vi "calculator.vi"() -> ()   [LabVIEW 2020]
panel:
  out "结果":string
  out "表达式":string
  in  "BACKPLACE":bool
  in  "C":bool
  in  "ln":bool
  in  "^":bool
  in  "tan":bool
  in  "cos":bool
  in  "sin":bool
  in  ")":bool
  in  "(":bool
  in  ".":bool
  in  "=":bool
  in  "0":bool
  in  "9":bool
  in  "8":bool
  in  "7":bool
  in  "6":bool
  in  "5":bool
  in  "4":bool
  in  "3":bool
  in  "2":bool
  in  "1":bool
  in  "÷":bool
  in  "×":bool
  in  "-":bool
  in  "+":bool
  # "科学计算器"
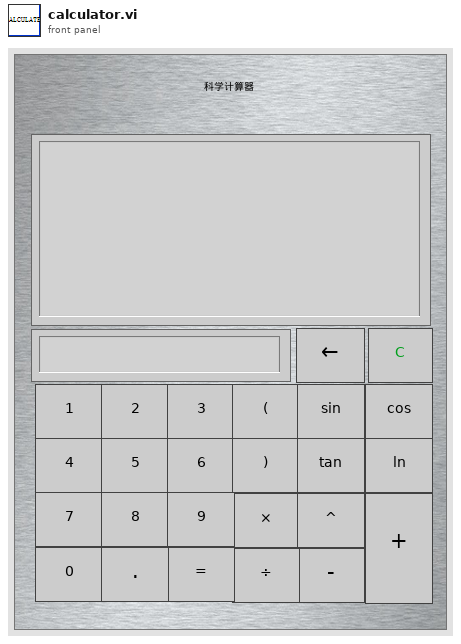
[diagram p1: front panel]
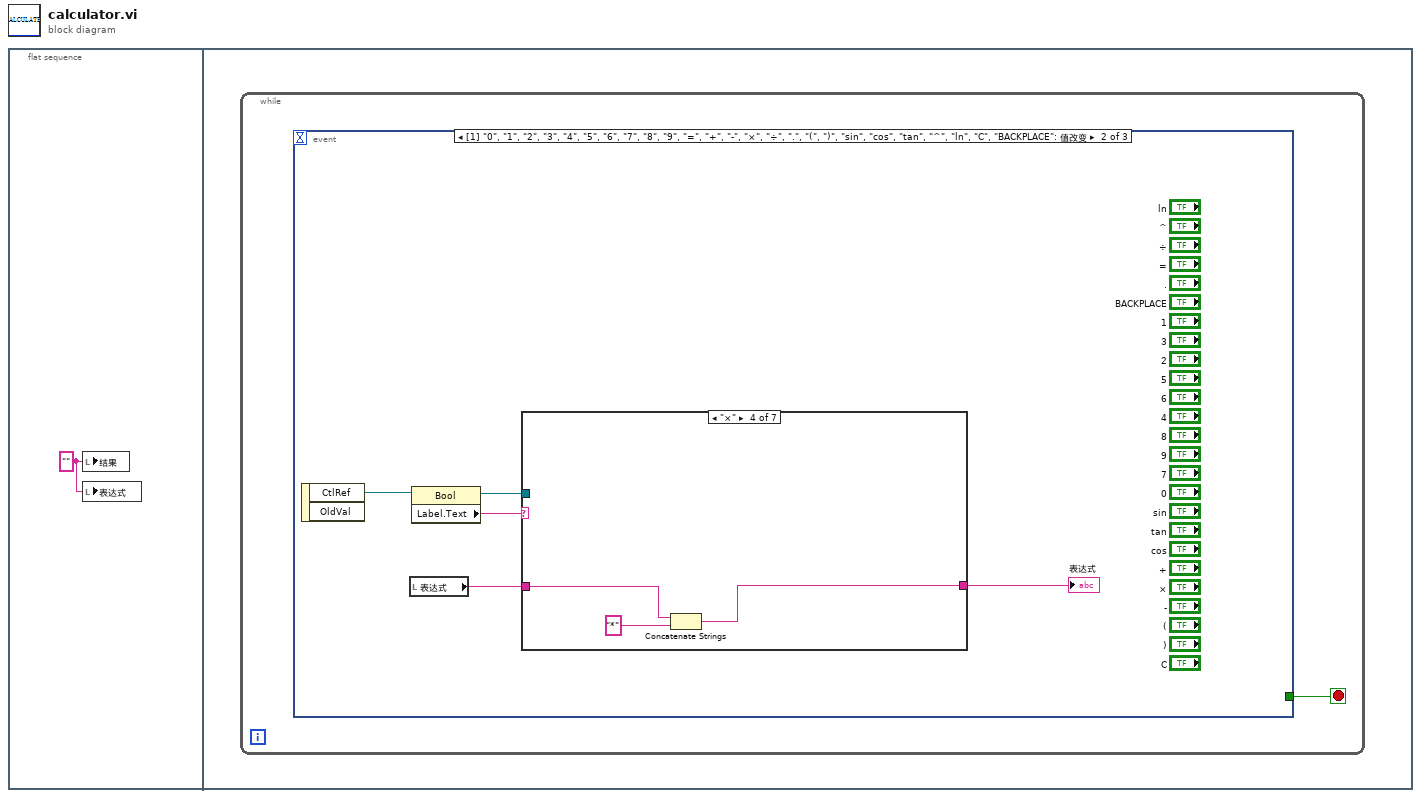
[diagram p0: block diagram]
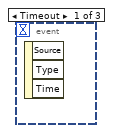
[diagram p2: hidden frame]
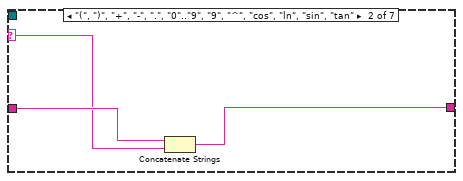
[diagram p4: hidden frame]
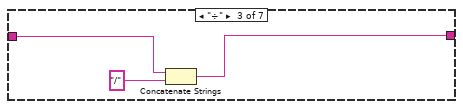
[diagram p5: hidden frame]
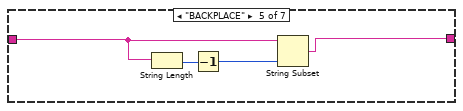
[diagram p6: hidden frame]
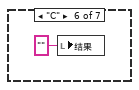
[diagram p7: hidden frame]
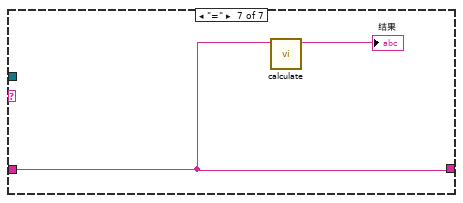
[diagram p8: hidden frame]
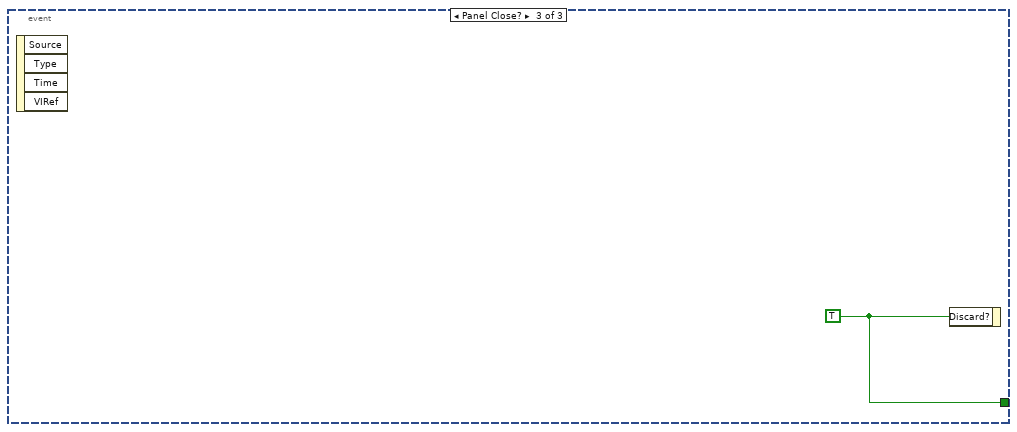
[diagram p9: hidden frame]
diagram:
  n1 = flat-sequence {
    frame #0 {
      w1 = "" ("结果")
      n2 = local write "结果"(w1) -> ()
      n3 = local write "表达式"(w1) -> ()
    }
    frame #1 {
      n4 = while {
        stop <- w2 stop-if-true
        n5 = event shown="[1] \"0\", \"1\", \"2\", \"3\", \"4\", \"5\", \"6\", \"7\", \"8\", \"9\", \"=\", \"+\", \"-\", \"×\", \"÷\", \".\", \"(\", \")\", \"sin\", \"cos\", \"tan\", \"^\", \"ln\", \"C\", \"BACKPLACE\": 值改变" {
          selector: _ -> [_ _ _]
          dyn-events: _ -> [_ _ _]
          timeout: _ -> [_ _ _]
          tunnel: [_ _ w25] -> w2
          event Timeout {
            n6 = event-data() -> ()  [unwired: 1 in, 3 out]
          }
          event "0", "1", "2", "3", "4", "5", "6", "7", "8", "9", "=", "+", "-", "×", "÷", ".", "(", ")", "sin", "cos", "tan", "^", "ln", "C", "BACKPLACE": Value Change {
            n7 = event-data() -> ("CtlRef"=w7:refnum<vi>)  [unwired: 1 in, 1 out]
            n8 = local read "表达式"() -> (w4:string)
            n9 = property class="Bool"(reference=w7) -> (reference out=w5:refnum<vi>, "Label.Text"=w6:string)  [unwired: 1 in, 1 out]
            n10 = case shown="\"×\"" w6 {
              selector: w6 -> [_ w9 _ _ _ _ _]
              tunnel: w5 -> [_ _ _ _ _ _ _]
              tunnel: [w8 w11 w14 w17 w21 _ w24] -> w3
              tunnel: w4 -> [w8 w10 w13 w16 w20 _ w24]
              frame "eee", Default {
              }
              frame "(", ")", "+", "-", ".", "0".."9", "9", "^", "cos", "ln", "sin", "tan" {
                n11 = Concatenate Strings(w10, w9) -> (w11:string)
              }
              frame "÷" {
                n12 = Concatenate Strings(w13, "/" ("字符串")) -> (w14:string)
              }
              frame "×" {
                n13 = Concatenate Strings(w16, "*" ("字符串")) -> (w17:string)
              }
              frame "BACKPLACE" {
                n14 = String Length(string=w20) -> (length=w19:i32)
                n15 = Decrement(x=w19) -> (x-1=w18:i32)
                n16 = String Subset(string=w20, length (rest)=w18) -> (substring=w21:string)  [unwired: 1 in]
              }
              frame "C" {
                n17 = local write "结果"("" ("结果")) -> ()
              }
              frame "=" {
                n18 = call "calculate.vi"("Formular"=w24) -> ("Result"=→"结果":string)  [unwired: 9 in, 1 out]
              }
            }
            "表达式" <- w3
          }
          event Panel Close? {
            w25 = TRUE ("放弃？")
            n19 = event-data() -> ()  [unwired: 1 in, 4 out]
            n20 = event-data("Discard?"=w25) -> ()  [unwired: 1 in, 1 out]
          }
        }
      }
    }
  }
